vi "usrp_rx.vi"() -> ()   [LabVIEW 2014]
uses:
  <vilib>/Analysis/baseanly.llb/Mean (DBL).vi
  <vilib>/addons/Modulation/Analog/support/mod_Set Error Source.vi
  var_rx_stop.vi
  <vilib>/addons/Modulation/Digital/Support/Common/Validators/mod_Generate Filter Coefficients Validate.vi
  <vilib>/addons/Modulation/Digital/General/subVIs/mod_Generate Filter Coefficients.vi
  <vilib>/imath/engines/lvmath2/RunTimeEngine/NodeEndStatement/NIMS_NodeEndStatement_Output.vi
  <instcachedir>/0/NIMS_NodeEndStatement_Output_53EC0D466D134D7ABD903AC30B43404B.lvgen/NIMS_NodeEndStatement_Output_53EC0D466D134D7ABD903AC30B43404B_001.vi
  <vilib>/imath/engines/lvmath2/RunTimeEngine/ErrorHandling/NIMS_Finalize Error.vi
  <instrlib>/niUSRP/niUSRP Fetch Rx Data (CDB Cluster).vi
  <vilib>/addons/Modulation/niDMT.lvlib
  <vilib>/Analysis/NI_AALBase.lvlib
panel:
  out "byte packets":cluster{string}[](array[cluster])
  out "Receive a packet":bool
  out "received power":dbl format="%0.6f"
  in  "PSK arity":enum16{"binary", "quadrature"}(ring)=enum."quadrature"
  in  "loop bandwidth":dbl=0.0314
  in  "nfilters":i32=32
  in  "samples per symbol":i32=4
  in  "stop":bool
  in  "number of samples":i64=20000
  in  "Configuration:Enabled Channels":string(combo)="0"
  in  "Clocking and Synchronization:Timebase Clock Source":string(combo)="Internal"
  in  "Clocking and Synchronization:Reference Frequency Source":string(combo)="Internal"
  out "coerced gain":dbl format="%#_6f"
  out "coerced carrier frequency":dbl=100000.0 format="%#_6p"
  out "coerced IQ rate":dbl=100000.0 format="%#_6p"
  in  "active antenna":string="RX2"
  in  "gain":dbl=10.0 format="%#_6f"
  in  "carrier frequency":dbl=915000000.0 format="%#_6p"
  in  "IQ rate":dbl=1000000.0 format="%#_6p"
  in  "device names":refnum<k15>="192.168.10.4"
  # "This is an USRP point-to-point link prototype\ndeveloped by Teng-Hui Huang. \nNetwork Information and Communications Laboratory, NTU Taiwan.\nThe prototype features implemented synchronization algorithms and \nphysical layer design which can be extended to applications such as\nvideo streaming or content delivery system.\n\nQuick start:\n1. Connect USRPs to PC\n2. Run \"usrp_tx.vi\"\n3. Run \"usrp_rx.vi\"\n4. Press \"Send text\" in usrp_tx.vi\nIf no error occurs, what you send will be shown in \"byte packets\" textbox\nFor any issues, please send me an e-mail\nhui811116@outlook.com\n\nThanks,\nTeng-Hui Huang"
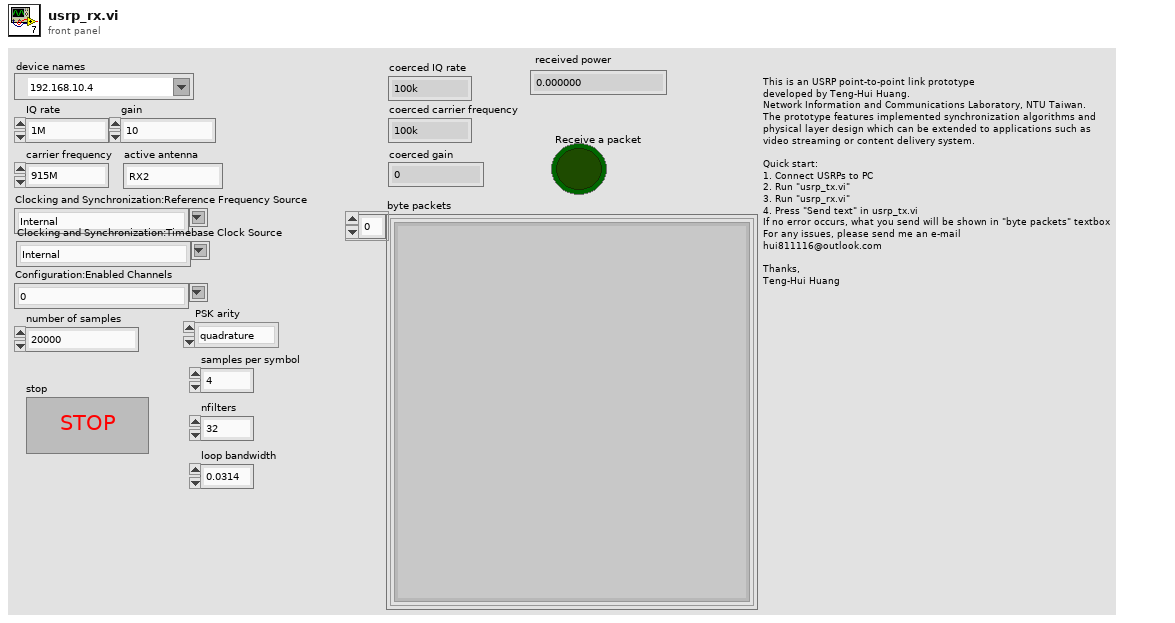
[diagram p1: front panel]
types:
  T1 = enum16{"none", "Raised Cosine", "Root Raised Cos", "Gaussian"}
  T2 = enum16{"FSK", "PSK", "QAM", "MSK", "PAM", "ASK", "CPM"}
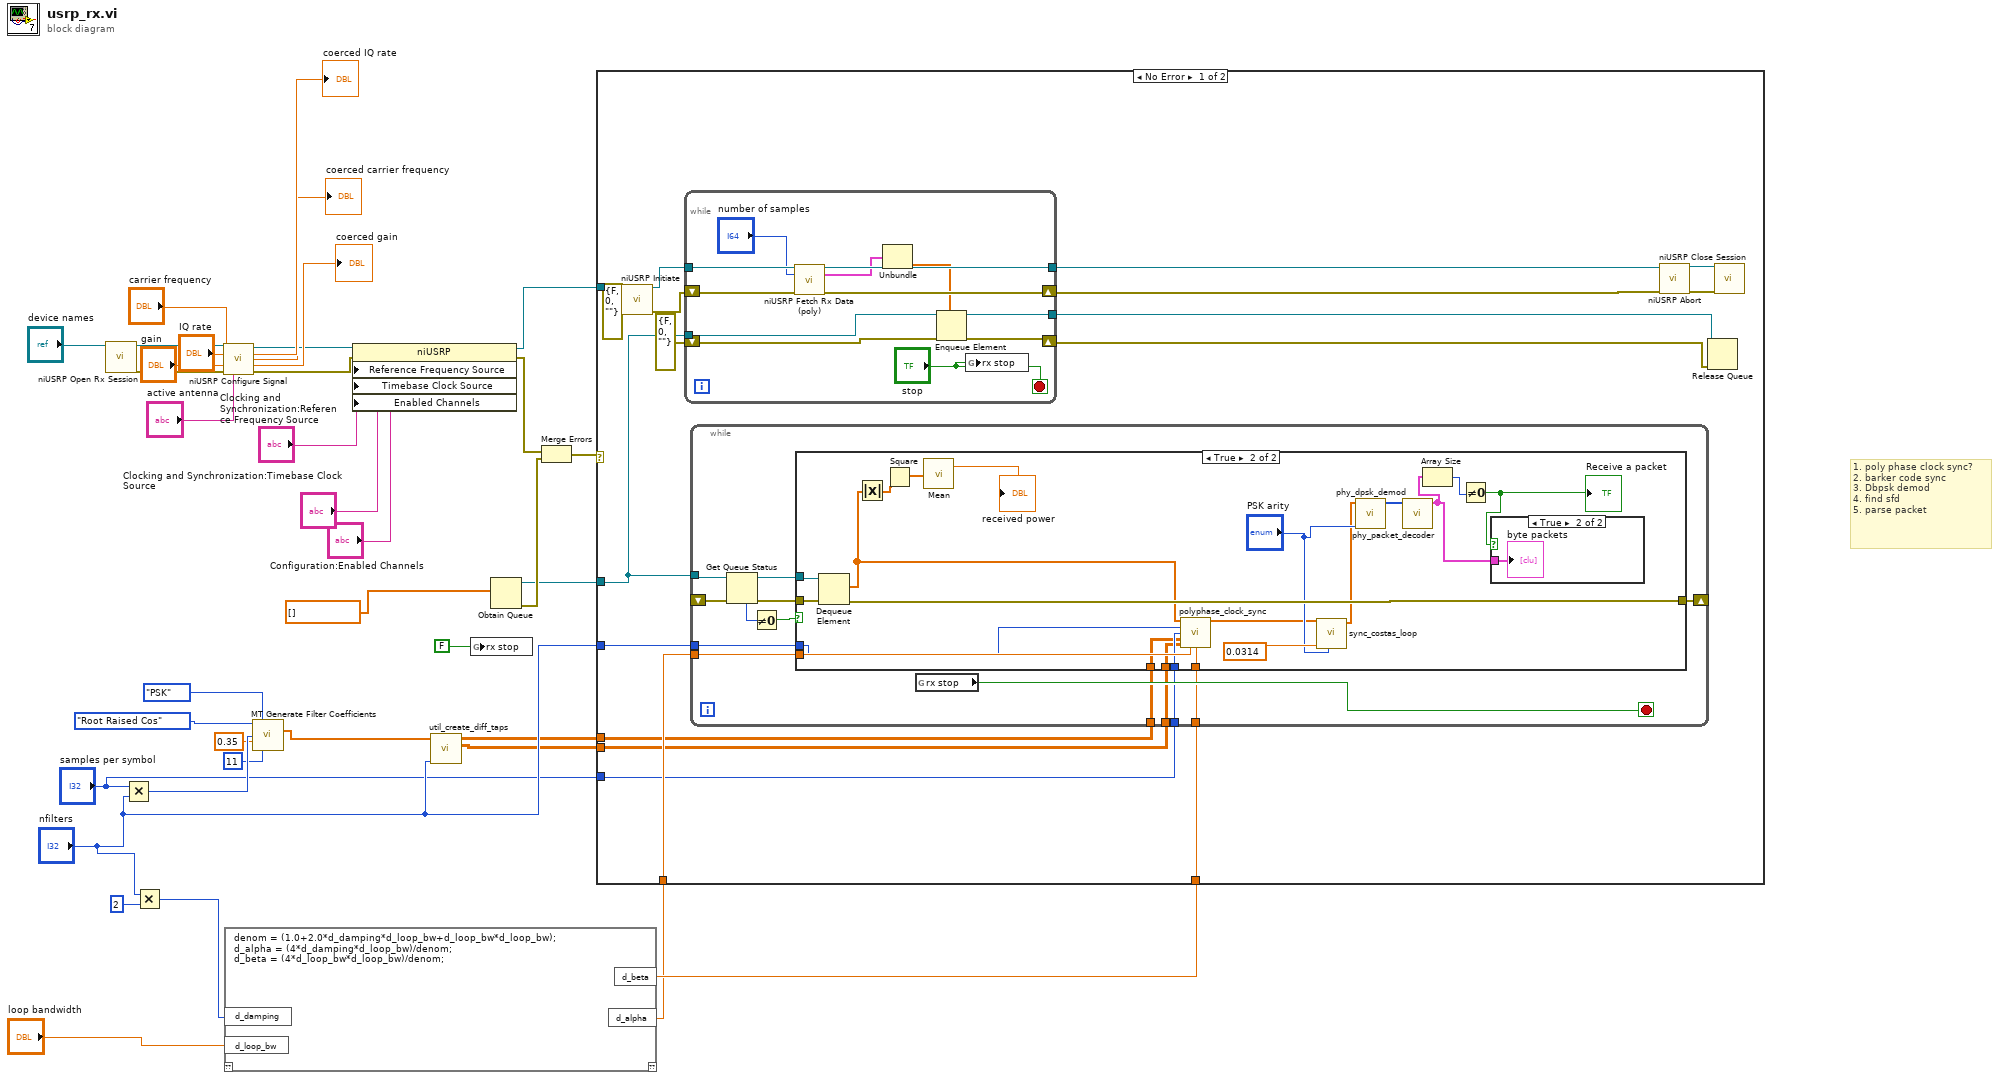
[diagram p0: block diagram]
diagram:
  # "1. poly phase clock sync?\n2. barker code sync\n3. Dbpsk demod\n4. find sfd\n5. parse packet"
  n1 = call <instrlib>:"niUSRP Open Rx Session.vi"("device names"="device names") -> ("session handle out"=w37:refnum<k15>, "error out"=w36:errorcluster)  [unwired: 13 in]
  n2 = Multiply(x="samples per symbol", y="nfilters") -> (x*y=w13:i32)
  n3 = Multiply(x="nfilters", y=2) -> (x*y=w8:i32)
  n4 = call <instrlib>:"niUSRP Configure Signal.vi"("session handle"=w37, "IQ rate"="IQ rate", "carrier frequency"="carrier frequency", "gain"="gain", "error in (no error)"=w36, "active antenna"="active antenna") -> ("session handle out"=w27:refnum<k15>, "coerced IQ rate"=→"coerced IQ rate":dbl, "coerced carrier frequency"=→"coerced carrier frequency":dbl, "coerced gain"=→"coerced gain":dbl, "error out"=w26:errorcluster)  [unwired: 5 in]
  n5 = mathscript code="denom = (1.0+2.0*d_damping*d_loop_bw+d_loop_bw*d_loop_bw);\nd_alpha = (4*d_damping*d_loop_bw)/denom;\nd_beta = (4*d_loop_bw*d_loop_bw)/denom;"("d_damping"=w8, "d_loop_bw"="loop bandwidth") -> ("d_alpha"=w5:dbl, "d_beta"=w6:dbl)  [unwired: 1 in, 1 out]
  n6 = call <vilib>:"MT Generate Filter Coefficients.vi"("pulse shaping filter (none)"=T1."Root Raised Cos", "modulation type"=T2."PSK", "matched samples per symbol (16)"=w13, "filter parameter"=0.35, "filter length (symbols)"=11) -> ("matched filter coefficients"=w10:dbl[])  [unwired: 8 in, 2 out]
  n7 = property class="niUSRP"(reference=w27, error in=w26, "Reference Frequency Source"="Clocking and Synchronization:Reference Frequency Source", "Timebase Clock Source"="Clocking and Synchronization:Timebase Clock Source", "Enabled Channels"="Configuration:Enabled Channels") -> (reference out=w22:refnum<k15>, error out=w18:errorcluster)
  n8 = call "util_create_diff_taps.vi"("nfilts"="nfilters", "taps"=w10) -> ("out diff taps"=w2:dbl[][], "out taps"=w1:dbl[][])  [unwired: 7 in, 1 out]
  n9 = global write "var_rx_stop.vi" "rx stop"(FALSE) -> ()
  n10 = Obtain Queue(element data type=cdb[] [] ("Y")) -> (queue out=w16:refnum<queue>, error out=w17:errorcluster)  [unwired: 4 in, 1 out]
  n11 = Merge Errors(w18, w17) -> (w19:errorcluster)
  n12 = case shown="No Error" w19 {
    tunnel: w22 -> [w49 _]
    tunnel: w16 -> [w47 _]
    tunnel: w6 -> [w43 _]
    tunnel: w5 -> [w42 _]
    tunnel: "nfilters" -> [w41 _]
    tunnel: "samples per symbol" -> [w40 _]
    tunnel: w1 -> [w39 _]
    tunnel: w2 -> [w38 _]
    frame No Error {
      n13 = call <instrlib>:"niUSRP Initiate.vi"("session handle"=w49, "error in (no error)"=errorcluster {"status"=FALSE, "code"=0, "source"=""}) -> ("session handle out"=w53:refnum<k15>, "error out"=w50:errorcluster)  [unwired: 12 in]
      n14 = while {
        tunnel: w53 -> [w104]
        shift-right: [w101] -> w51
        shift-left: w50 -> [w103]
        tunnel: [w100] -> w52
        tunnel: w47 -> [w96]
        shift-right: [w95] -> w45
        shift-left: errorcluster {"status"=FALSE, "code"=0, "source"=""} ("error out") -> [w94]
        tunnel: [w93] -> w44
        stop <- "stop" stop-if-true
        n15 = call-poly <instrlib>:"niUSRP Fetch Rx Data (poly).vi"("session handle"=w104, "number of samples"="number of samples", "error in (no error)"=w103) -> ("session handle out"=w100:refnum<k15>, "data"=w98:cluster{"t0":dbl, "dt":dbl, "Y":cdb[]}, "error out"=w101:errorcluster)  [unwired: 9 in, 1 out]
        n16 = Unbundle(w98) -> ("Y"=w97:cdb[])  [unwired: 2 out]
        n17 = Enqueue Element(queue=w96, element=w97, error in (no error)=w94) -> (queue out=w93:refnum<queue>, error out=w95:errorcluster)  [unwired: 1 in, 1 out]
        n18 = global write "var_rx_stop.vi" "rx stop"("stop") -> ()
      }
      n19 = while {
        tunnel: w47 -> [w68]
        shift-right: [w62] -> _
        shift-left: _ -> [w63]
        tunnel: w43 -> [w61]
        tunnel: w42 -> [w60]
        tunnel: w41 -> [w59]
        tunnel: w40 -> [w58]
        tunnel: w39 -> [w57]
        tunnel: w38 -> [w56]
        stop <- w69 stop-if-true
        n20 = Get Queue Status(queue=w68, error in (no error)=w63) -> (queue out=w65:refnum<queue>, error out=w64:errorcluster, # elements in queue=w67:i32)  [unwired: 1 in, 5 out]
        n21 = Not Equal To 0?(x=w67) -> (x != 0?=w66:bool)
        n22 = case shown="True" w66 {
          tunnel: w65 -> [_ w91]
          tunnel: w64 -> [w70 w90]
          tunnel: [w70 w89] -> w62
          tunnel: w61 -> [_ w88]
          tunnel: w60 -> [_ w87]
          tunnel: w59 -> [_ w86]
          tunnel: w58 -> [_ w85]
          tunnel: w57 -> [_ w84]
          tunnel: w56 -> [_ w83]
          frame False {
          }
          frame True {
            n23 = Dequeue Element(queue=w91, error in (no error)=w90) -> (element=w72:cdb[], error out=w89:errorcluster)  [unwired: 1 in, 2 out]
            n24 = Absolute Value(x=w72) -> (abs(x)=w81:dbl[])
            n25 = Square(x=w81) -> (x^2=w80:dbl[])
            n26 = call-poly <vilib>:"Mean.vi"("X"=w80) -> ("mean"=→"received power":dbl)  [unwired: 1 out]
            n27 = call "polyphase_clock_sync.vi"("samples"=w72, "nfilts"=w86, "sps"=w85, "taps"=w84, "diff taps"=w83, "alpha"=w87, "beta"=w88) -> ("out symbols"=w73:cdb[])  [unwired: 7 in, 1 out]
            n28 = call "sync_costas_loop.vi"("arity"="PSK arity", "loop bandwidth"=0.0314, "symbols"=w73) -> ("outputs"=w71:cdb[])  [unwired: 8 in]
            n29 = call "phy_dpsk_demod.vi"("arity"="PSK arity", "dpsk"=w71) -> ("bitstream"=w77:u8[])  [unwired: 9 in]
            n30 = call "phy_packet_decoder.vi"("bits"=w77) -> ("bytes cluster"=w74:cluster{string}[])  [unwired: 10 in]
            n31 = Array Size(array=w74) -> (size(s)=w76:i32)
            n32 = Not Equal To 0?(x=w76) -> (x != 0?=w75:bool)
            "Receive a packet" <- w75
            n33 = case shown="True" w75 {
              tunnel: w74 -> [_ w92]
              frame False {
              }
              frame True {
                "byte packets" <- w92
              }
            }
          }
        }
        n34 = global read "var_rx_stop.vi" "rx stop"() -> (w69:bool)
      }
      n35 = call <instrlib>:"niUSRP Abort.vi"("session handle"=w52, "error in (no error)"=w51) -> ("session handle out"=w55:refnum<k15>, "error out"=w54:errorcluster)  [unwired: 12 in]
      n36 = Release Queue(queue=w44, error in (no error)=w45) -> ()  [unwired: 1 in, 3 out]
      n37 = call <instrlib>:"niUSRP Close Session.vi"("session handle"=w55, "error in (no error)"=w54) -> ()  [unwired: 13 in, 1 out]
    }
    frame Error {
    }
  }
